vi "Sprite_GetSprites.vi"(11 "Sprite Path":path) -> (3 "Sprites":u8[](array[numeric]))   [LabVIEW 2020]
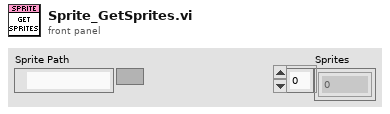
[diagram p1: front panel]
types:
  T1 = typedef "imagedata.ctl" = cluster{"image type":i32, "image depth":i32, "image":u8[], "mask":u8[], "colors":u32[], "Rectangle":cluster{"left":i16, "top":i16, "right":i16, "bottom":i16}}
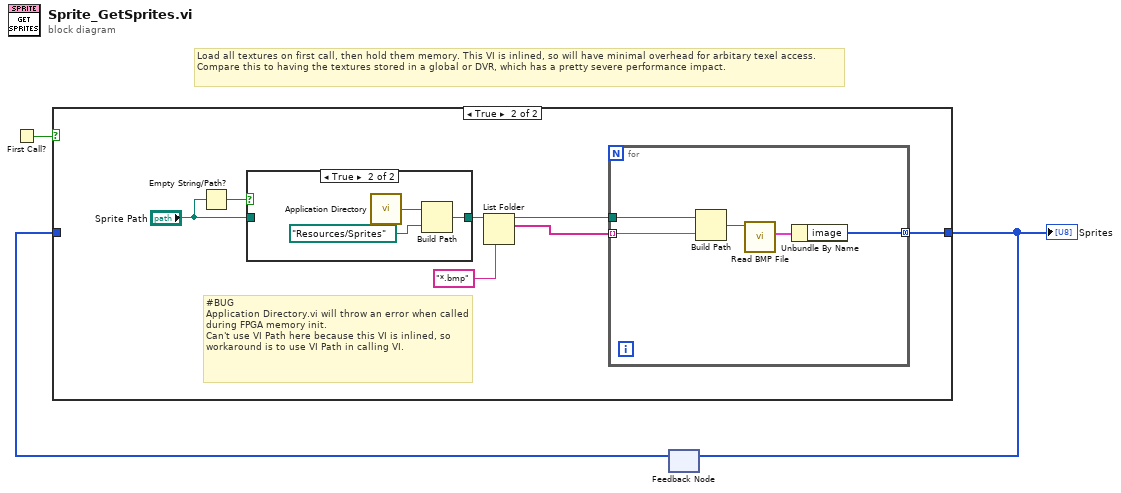
[diagram p0: block diagram]
diagram:
  # "Load all textures on first call, then hold them memory. This VI is inlined, so will have minimal overhead for arbitary texel access. Compare this to having the textures stored in a global or DVR, which has a pretty severe performance impact."
  n1 = First Call?() -> (First Call?: T/F=w3:bool)
  n2 = feedback #1() -> (w2:u8[])  [unwired: 1 in]
  n3 = case shown="True" w3 {
    tunnel: [w4 w11] -> w1
    tunnel: w2 -> [w4 _]
    frame False {
    }
    frame True {
      # "#BUG\nApplication Directory.vi will throw an error when called during FPGA memory init.\nCan't use VI Path here because this VI is inlined, so workaround is to use VI Path in calling VI."
      n4 = Empty String/Path?(string/path="Sprite Path") -> (empty?=w7:bool)
      n5 = case shown="True" w7 {
        tunnel: [w12 w14] -> w8
        tunnel: "Sprite Path" -> [w12 _]
        frame False {
        }
        frame True {
          n6 = call <vilib>:"Application Directory.vi"() -> ("Application Directory"=w13:path)
          n7 = Build Path(base path=w13, name or relative path=path "Resources/Sprites") -> (appended path=w14:path)
        }
      }
      n8 = List Folder(path=w8, pattern="*.bmp") -> (path out=w9:path, filenames=w5:string[])  [unwired: 2 in, 2 out]
      n9 = for {
        tunnel: w5 -> [w20] mode=indexing
        tunnel: [w19] -> w11 mode=concatenating
        tunnel: w9 -> [w18]
        n10 = Build Path(base path=w18, name or relative path=w20) -> (appended path=w17:path)
        n11 = call <vilib>:"Read BMP File.vi"("path to BMP file"=w17) -> ("image data"=w16:T1)  [unwired: 8 in, 2 out]
        n12 = Unbundle By Name(w16) -> ("image"=w19:u8[])
      }
    }
  }
  "Sprites" <- w1
  n13 = feedback-in #1(w1) -> ()
